vi "StartLock.vi"(0 "VISA resource name":refnum<visa-resource-name>, 5 "Input channel":T2, 7 "Output channel":T1, 9 "Lock settings":T3={"K / V/V"=0.0, "T_I / s"=0.0, "T_D / s"=0.0, "Target Error / V"=0.0, "N"=10.0}, 11 "error in (no error)":errorcluster) -> (4 "VISA resource name out":refnum<visa-resource-name>, 8 "PID settings confirmation":string, 15 "error out":errorcluster)   [LabVIEW 2015, in "YbTempCtrl.lvlib"]
doc: "Start a PID lock with the given settings"
uses:
  YbTempCtrl.lvlib
  Typedefs/InputChannelTypedef.ctl
  Typedefs/OutputChannelTypedef.ctl
panel:
  out "Config string":string
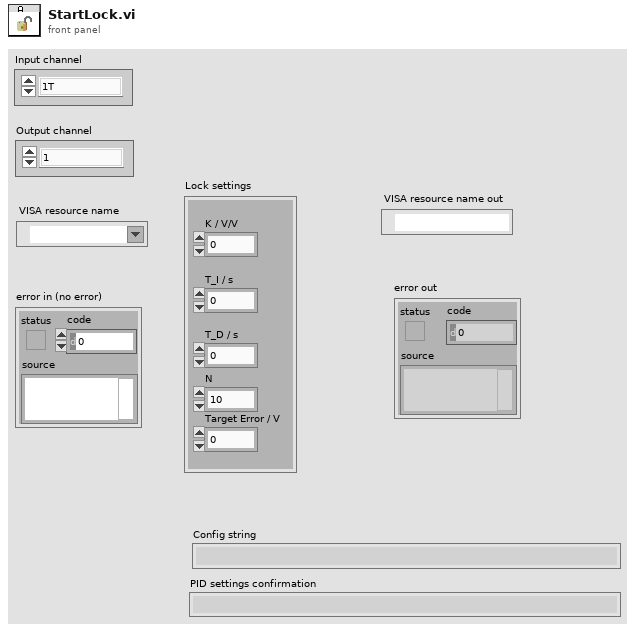
[diagram p1: front panel]
types:
  T1 = typedef "YbTempCtrl.lvlib/OutputChannelTypedef.ctl" = enum16{"1", "2", "3", "4", "BPA", "BPB"}
  T2 = typedef "YbTempCtrl.lvlib/InputChannelTypedef.ctl" = enum16{"1T", "2T", "TMP", "POW"}
  T3 = cluster{"K / V/V":dbl, "T_I / s":dbl, "T_D / s":dbl, "Target Error / V":dbl, "N":dbl}
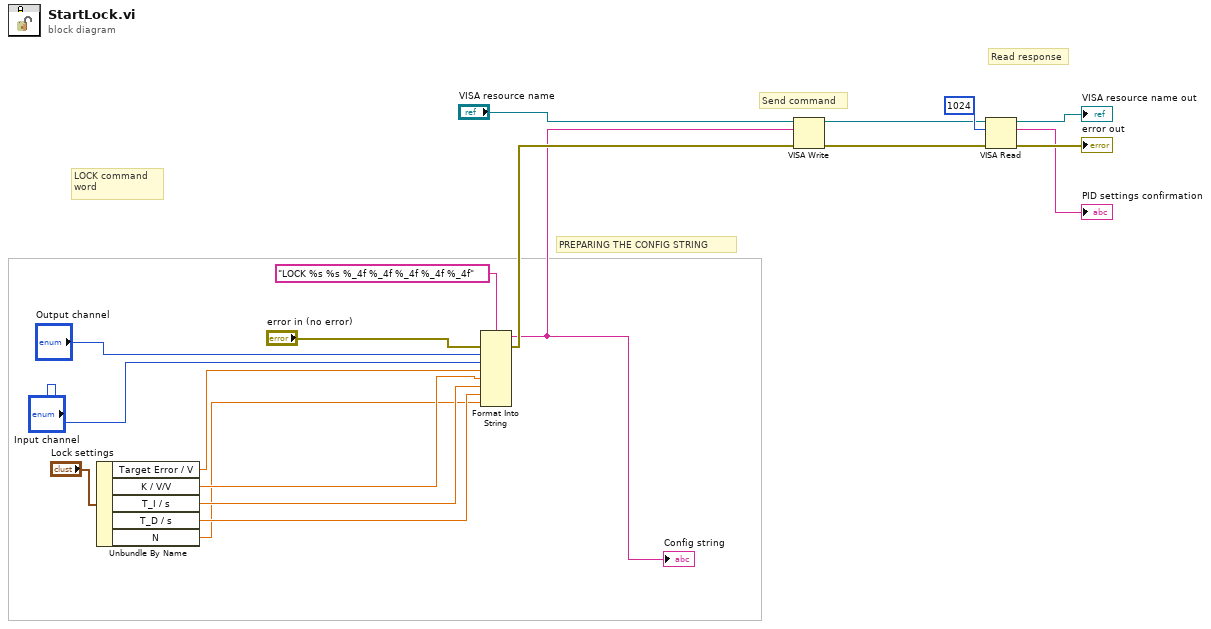
[diagram p0: block diagram]
diagram:
  # "Read response"
  # "Send command"
  # "PREPARING THE CONFIG STRING"
  # "LOCK command\nword"
  n1 = Unbundle By Name("Lock settings") -> ("Target Error / V"=w7:dbl, "K / V/V"=w6:dbl, "T_I / s"=w5:dbl, "T_D / s"=w4:dbl, "N"=w3:dbl)
  n2 = Format Into String(format string="LOCK %s %s %_4f %_4f %_4f %_4f %_4f", error in="error in (no error)", "Output channel", "Input channel", w7, w6, w5, w4, w3) -> (resulting string=w10:string, error out=w16:errorcluster)  [unwired: 1 in]
  "Config string" <- w10
  n3 = VISA Write(VISA resource name="VISA resource name", write buffer=w10, error in (no error)=w16) -> (VISA resource name out=w9:refnum<visa-resource-name>, error out=w8:errorcluster)  [unwired: 1 out]
  n4 = VISA Read(VISA resource name=w9, byte count=u32 1024, error in (no error)=w8) -> (VISA resource name out=→"VISA resource name out":refnum<visa-resource-name>, read buffer=→"PID settings confirmation":string, error out=→"error out":errorcluster)  [unwired: 1 out]
